vi "Receive Authorization Request.vi"(8 "error in (no error)":errorcluster, 11 "Connection in":refnum<class "Connection.lvclass">) -> (0 "error out":errorcluster, 1 "auth packet received":bool, 2 "Authorization":T1, 3 "Connection out":refnum<class "Connection.lvclass">, 4 "timed out":bool)   [LabVIEW 2013, in "Connection_GOSPL.lvlib" / "Connection.lvclass"]
uses:
  Connection.lvclass
  auth -- cluster.ctl
  Connection.lvclass/Connection.ctl
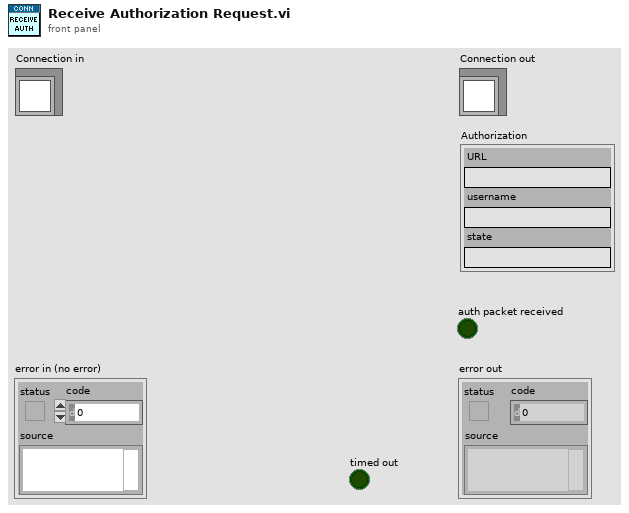
[diagram p1: front panel]
types:
  T1 = typedef "Connection_GOSPL.lvlib/Connection.lvclass/auth -- cluster.ctl" = cluster{"URL":string, "username":string, "state":string}
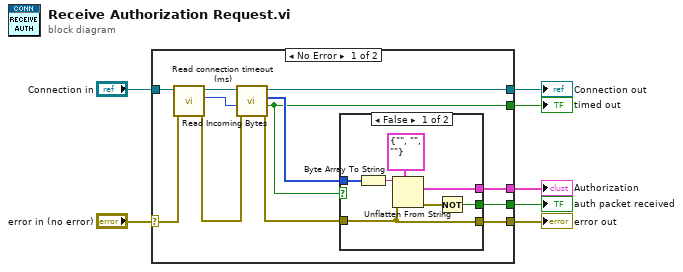
[diagram p0: block diagram]
diagram:
  n1 = case shown="No Error" "error in (no error)" {
    selector: "error in (no error)" -> [w13 w29]
    tunnel: [w12 w29] -> w6
    tunnel: [w16 w28] -> w4
    tunnel: "Connection in" -> [w18 w28]
    tunnel: [w10 _] -> w3
    tunnel: [w9 _] -> w2
    tunnel: [w8 _] -> w1
    frame No Error {
      n2 = call "Read connection timeout (ms).vi"("error in (no error)"=w13, "Connection in"=w18) -> ("error out"=w14:errorcluster, "connection timeout (ms)"=w15:i32, "Connection out"=w17:refnum<class "Connection.lvclass">)  [unwired: 7 in]
      n3 = call-dynamic "Read Incoming Bytes.vi"("error in (no error)"=w14, "timeout (1000 ms)"=w15, "Connection in"=w17) -> ("error out"=w11:errorcluster, "timed out"=w9:bool, "Bytes"=w19:u8[], "Connection out"=w16:refnum<class "Connection.lvclass">)  [unwired: 4 in, 1 out]
      n4 = case shown="False" w9 {
        tunnel: w19 -> [w24 _]
        tunnel: [w22 w27] -> w12
        tunnel: w11 -> [w22 w27]
        tunnel: [w23 _] -> w10
        tunnel: [w20 _] -> w8
        frame False {
          n5 = Byte Array To String(unsigned byte array=w24) -> (string=w25:string)
          n6 = Unflatten From String(type=T1 {"URL"="", "username"="", "state"=""} ("Authentication"), binary string=w25, error in (no error)=w22) -> (value=w23:T1, error out=w21:errorcluster)  [unwired: 2 in, 1 out]
          n7 = Not(x=w21) -> (.not. x?=w20:bool)
        }
        frame True {
        }
      }
    }
    frame Error {
    }
  }
  "error out" <- w6
  "Connection out" <- w4
  "Authorization" <- w3
  "timed out" <- w2
  "auth packet received" <- w1
